vi "TrapTest-2017-06-02.vi"() -> ()   [LabVIEW 2010]
uses:
  <vilib>/userDefined/High Color/nirio_resource_hc.ctl
  <vilib>/rvi/interface/nirviOpenFPGA/nirviOpenFPGA.xnode
  C:/Users/HAGAR-IV/Desktop/Zeugs/markus/version feb 2012/FPGA Bitfiles/pertrasgcfpga2_FPGATarget_Trap1-02-06-2017_6789B2A8.lvbitx
  C:/Users/HAGAR-IV/Desktop/Zeugs/Johnny/pertrasgc fpga/Trap1-02-06-2017.vi
  <vilib>/rvi/ClientSDK/nirviWhatTheDeviceIsDoing.ctl
  <vilib>/rvi/interface/nirviReadWriteControl/nirviReadWriteControl.xnode
  <vilib>/rvi/interface/common/niFpgaNodeNameForErrorReporting.ctl
  <vilib>/rvi/errors/niLvFpgaWhatHappensToTopLevelVI.ctl
  <vilib>/rvi/interface/nirviMethod/nirviMethod.xnode
  <vilib>/rvi/interface/nirviCloseFPGA/nirviCloseFPGA.xnode
  <vilib>/FPGAPlugInAG/cRIO-9114/niLvFpga_Open_cRIO-9114.vi
  <vilib>/rvi/interface/common/dynamic/niFpgaDynamicAddResources.vi
  <vilib>/Utility/error.llb/Error Cluster From Error Code.vi
  <vilib>/rvi/errors/niLvFpgaAdjustHostInterfaceError.vi
  <vilib>/FPGAPlugInAG/Dynamic/niLvFpga_Close_Dynamic.vi
  NiFpgaLv.dll
panel:
  in  "Bumm!":dbl
  in  "knallen!":bool
  out "t3":u32
  out "U":dbl
  in  "d1":dbl
  out "dt/t":dbl
  out "R":dbl
  in  "d0":dbl
  out "T":dbl
  in  "tau":dbl
  in  "heizen":bool
  in  "t1(us)":u16
  in  "t0(us)":u16
  in  "Löschen":bool
  out "Waveform Graph":dbl[](graph)
  in  "stop":bool
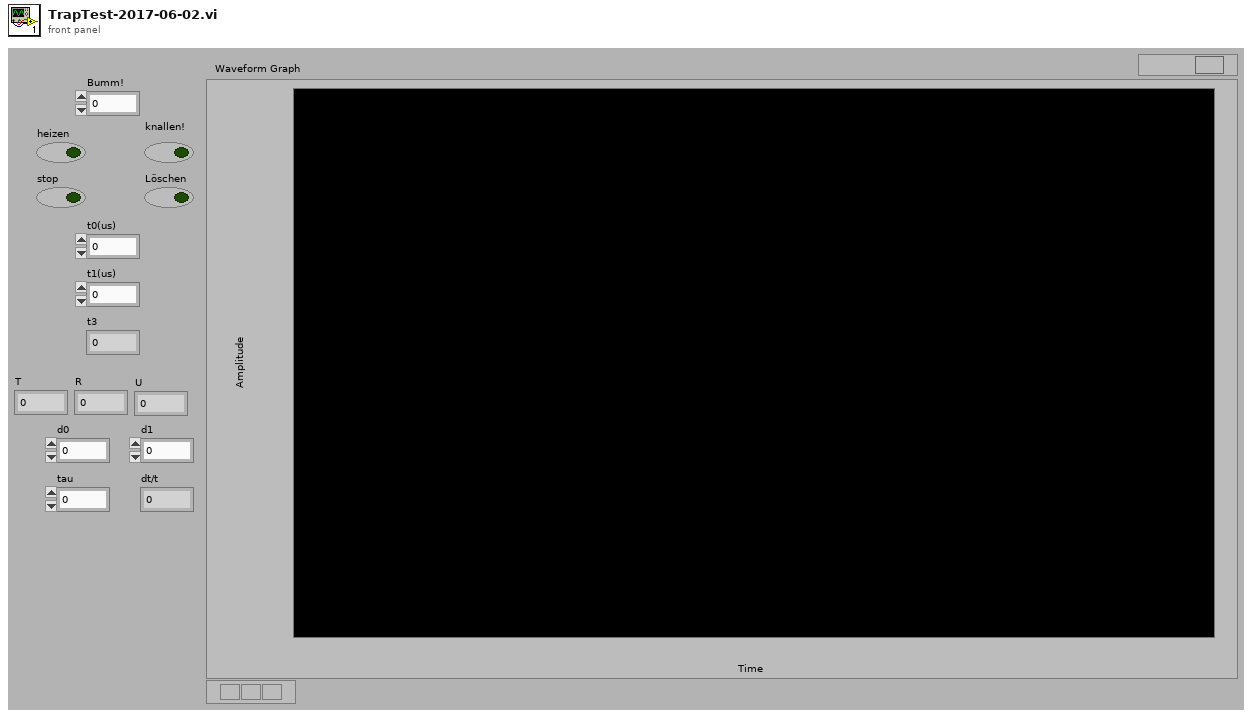
[diagram p1: front panel]
types:
  T1 = typedef "niFpgaNodeNameForErrorReporting.ctl" = enum16{"Open FPGA VI Reference", "Read/Write Control", "Invoke Method: Abort", "Invoke Method: Acknowledge IRQ", "Invoke Method: Download", "Invoke Method: FIFO.Configure", "Invoke Method: FIFO.Read", "Invoke Method: FIFO.Start", "Invoke Method: FIFO.Stop", "Invoke Method: FIFO.Write", "Invoke Method: Reset", "Invoke Method: Run", "Invoke Method: Wait on IRQ", "Close FPGA VI Reference"}
  T2 = typedef "niLvFpgaWhatHappensToTopLevelVI.ctl" = enum16{"top level VI scripted behind XNode", "top level VI inlined behind XNode"}
  T3 = typedef "nirviWhatTheDeviceIsDoing.ctl" = enum32{"nothing", "something other than LabVIEW FPGA", "FPGA interface", "interactive", "emulation"}
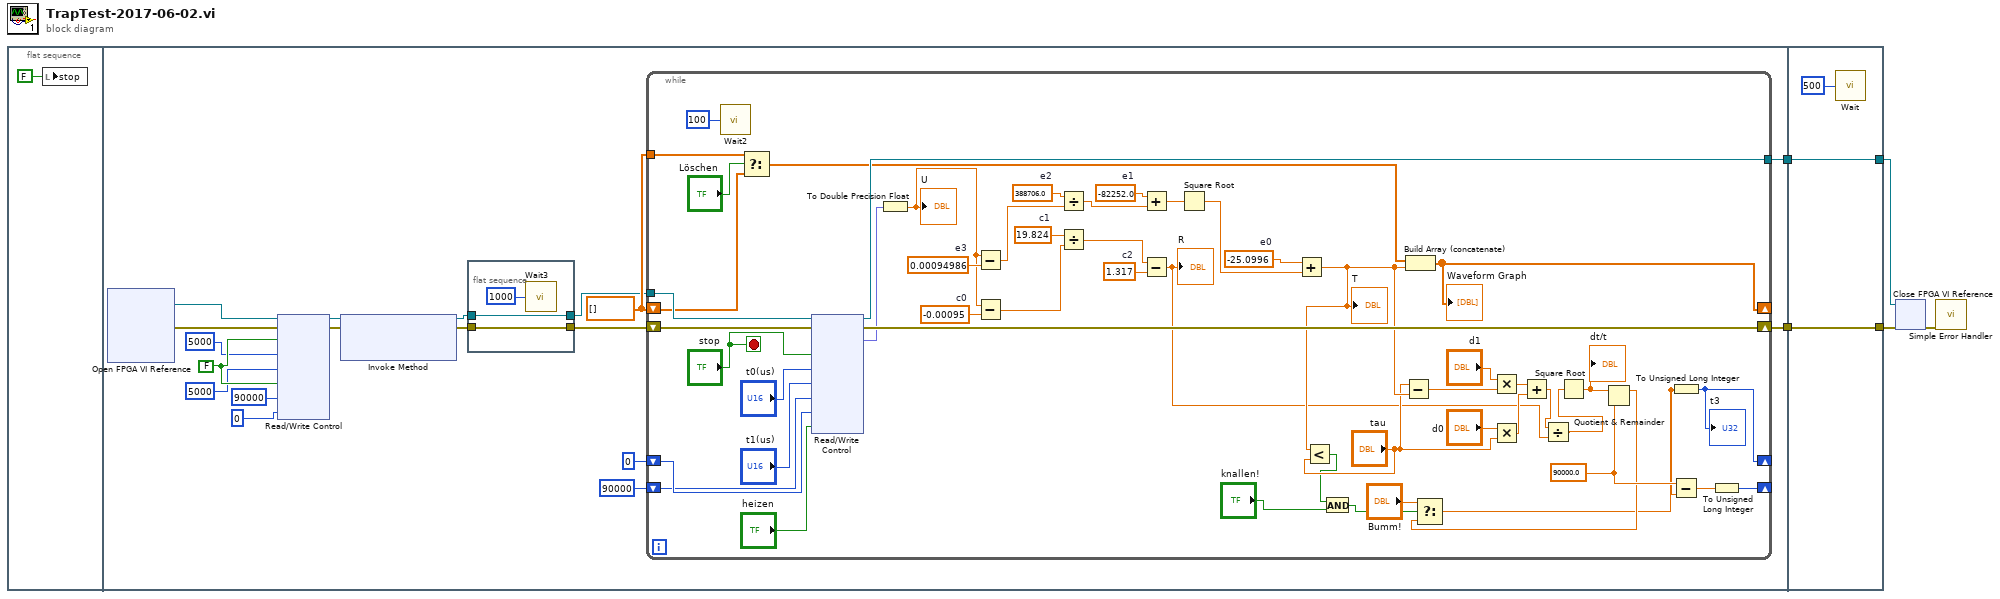
[diagram p0: block diagram]
diagram:
  n1 = flat-sequence {
    tunnel: [w20] -> w5
    tunnel: [w19] -> w3
    tunnel: w5 -> [w498]
    tunnel: [w498] -> w4
    tunnel: w3 -> [w497]
    tunnel: [w497] -> w2
    frame #0 {
      n2 = local write "stop"(FALSE ("stop")) -> ()
    }
    frame #1 {
      w18 = dbl[] []
      w15 = FALSE ("stop")
      n3 = xnode "Open FPGA VI Reference"() -> ("FPGA VI Reference Out"=w24:refnum<k20>, "error out"=w23:errorcluster)  [unwired: 2 in]
      n4 = xnode "Read/Write Control"("FPGA VI Reference In"=w24, "error in"=w23, "stop"=w15, "t0(ms)"=u16 5000, "t1(ms)"=u16 5000, "heizen"=w15, "t2(ms)"=u32 90000, "t3(ms)"=u32 0) -> ("FPGA VI Reference Out"=w22:refnum<k20>, "error out"=w21:errorcluster)
      n5 = xnode "Invoke Method"("FPGA VI Reference In"=w22, "error in"=w21) -> ("FPGA VI Reference Out"=w10:refnum<k20>, "error out"=w8:errorcluster)  [unwired: 1 in]
      n6 = flat-sequence {
        tunnel: w10 -> [w27]
        tunnel: [w27] -> w9
        tunnel: w8 -> [w26]
        tunnel: [w26] -> w7
        frame #0 {
          n7 = call "Wait3"("Count(mSec)"=u32 1000) -> ()  [unwired: 1 out]
        }
      }
      n8 = while {
        tunnel: w9 -> [w79]
        shift-right: [w77] -> _
        shift-left: w18 -> [w73]
        tunnel: [w76] -> w20
        shift-right: [w75] -> w19
        shift-left: w7 -> [w78]
        tunnel: w18 -> [w71]
        shift-right: [w48] -> _
        shift-left: u32 0 -> [w47]
        shift-right: [w44] -> _
        shift-left: u32 90000 -> [w43]
        stop <- "stop" stop-if-true
        w46 = 90000.0 ("y")
        w50 = 1.317  # c2
        w53 = 19.824  # c1
        w54 = -0.00095  # c0
        w65 = 0.00094986  # e3
        w63 = 388706.0  # e2
        w60 = -82252.0  # e1
        w58 = -25.0996  # e0
        n9 = call "Wait2"("Count(mSec)"=u32 100) -> ()  [unwired: 1 out]
        n10 = Select(t=w71, s="Löschen", f=w73) -> (s? t:f=w72:dbl[])
        n11 = xnode "Read/Write Control"("FPGA VI Reference In"=w79, "error in"=w78, "stop"="stop", "t0(ms)"="t0(us)", "t1(ms)"="t1(us)", "t2(ms)"=w43, "t3(ms)"=w47, "heizen"="heizen") -> ("FPGA VI Reference Out"=w76:refnum<k20>, "error out"=w75:errorcluster, "U"=w64:fxp<+/-,26,5>)
        n12 = To Double Precision Float(number=w64) -> (double precision float=w55:dbl)
        "U" <- w55
        n13 = Subtract(x=w55, y=w65) -> (x-y=w62:dbl)
        n14 = Subtract(x=w55, y=w54) -> (x-y=w52:dbl)
        n15 = Divide(x=w63, y=w62) -> (x/y=w61:dbl)
        n16 = Divide(x=w53, y=w52) -> (x/y=w51:dbl)
        n17 = Add(x=w60, y=w61) -> (x+y=w59:dbl)
        n18 = Subtract(x=w51, y=w50) -> (x-y=w33:dbl)
        "R" <- w33
        n19 = Square Root(x=w59) -> (sqrt(x)=w57:dbl)
        n20 = Add(x=w58, y=w57) -> (x+y=w39:dbl)
        "T" <- w39
        n21 = Less?(x=w39, y="tau") -> (x < y?=w37:bool)
        n22 = And(x=w37, y="knallen!") -> (x .and. y?=w32:bool)
        n23 = Subtract(x="tau", y=w39) -> (x-y=w42:dbl)
        n24 = Build Array (concatenate)(w72, w39) -> (w77:dbl[])
        "Waveform Graph" <- w77
        n25 = Multiply(x="d1", y=w42) -> (x*y=w40:dbl)
        n26 = Multiply(x="d0", y="tau") -> (x*y=w35:dbl)
        n27 = Add(x=w40, y=w35) -> (x+y=w34:dbl)
        n28 = Divide(x=w34, y=w33) -> (x/y=w28:dbl)
        n29 = Square Root(x=w28) -> (sqrt(x)=w49:dbl)
        "dt/t" <- w49
        n30 = Quotient & Remainder(x=w49, y=w46) -> (x-y*floor(x/y)=w31:dbl)  [unwired: 1 out]
        n31 = Select(t="Bumm!", s=w32, f=w31) -> (s? t:f=w30:dbl)
        n32 = To Unsigned Long Integer(number=w30) -> (unsigned 32bit integer=w48:u32)
        "t3" <- w48
        n33 = Subtract(x=w46, y=w30) -> (x-y=w45:dbl)
        n34 = To Unsigned Long Integer(number=w45) -> (unsigned 32bit integer=w44:u32)
      }
    }
    frame #2 {
      n35 = call "Wait"("Count(mSec)"=u32 500) -> ()  [unwired: 1 out]
    }
  }
  n36 = xnode "Close FPGA VI Reference"("FPGA VI Reference In"=w4, "error in"=w2) -> ("error out"=w1:errorcluster)
  n37 = call <vilib>:"Simple Error Handler.vi"("error in (no error)"=w1) -> ()  [unwired: 4 in, 5 out]
